vi "asset.create_commit.vi"(8 "error in":errorcluster, 11 "AssetCreateStaging in":refnum<class "AssetCreateStaging.lvclass">) -> (0 "error out":errorcluster, 3 "AssetCreateStaging out":refnum<class "AssetCreateStaging.lvclass">)   [LabVIEW 2020, in "AssetCreateStaging.lvclass"]
doc: "Creates the staged asset in Nominal and returns a handle to it."
uses:
  AssetCreateStaging.lvclass
  AssetCreateStaging.lvclass/AssetCreateStaging.ctl
  client.lvlib
panel:
  out "out_asset out":i32
  in  "staging":i32
  in  "out_asset":i32
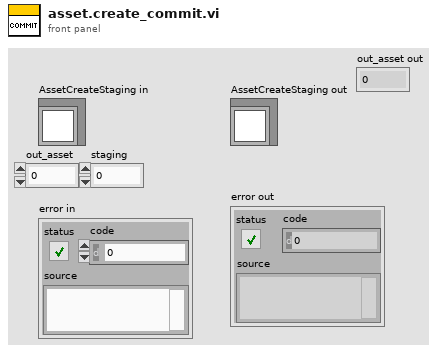
[diagram p1: front panel]
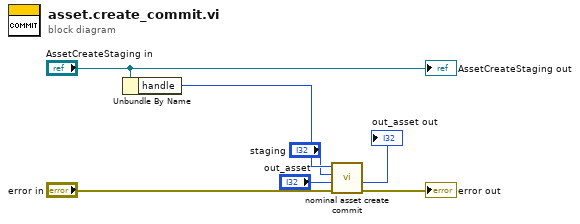
[diagram p0: block diagram]
diagram:
  n1 = Unbundle By Name("AssetCreateStaging in") -> ("handle"=w5:i32)
  n2 = call "nominal asset create commit.vi"("error in (no error)"="error in", "out_asset"="out_asset", "staging"="staging", "client"=w5) -> ("error out"=→"error out":errorcluster, "out_asset out"=→"out_asset out":i32)  [unwired: 5 in, 1 out]
  "AssetCreateStaging out" <- "AssetCreateStaging in"
